vi "layout.vi"(0 "reference":refnum<class "ImplicitParameterNode.lvclass">, 1 "graph":refnum<class "Graph.lvclass">, 2 "graphics":refnum<class "Graphics.lvclass">, 3 "grid":refnum<class "Grid.lvclass">, 5 "error in (no error)":errorcluster) -> (14 "reference out":refnum<class "ImplicitParameterNode.lvclass">, 19 "error out":errorcluster)   [LabVIEW 2014, in "ImplicitParameterNode.lvclass"]
doc: "public void layout(Graph g, Graphics2D g2, Grid grid)"
uses:
  <resource>/Framework/Providers/Open_GDS/UML/ImplicitParameterNode_class/ImplicitParameterNode.lvclass
  <resource>/Framework/Providers/Open_GDS/UML/Graph_class/Graph.lvclass
  <resource>/Framework/Providers/Open_GDS/UML/Graphics_class/Graphics.lvclass
  <resource>/Framework/Providers/Open_GDS/UML/Grid_class/Grid.lvclass
  <resource>/Framework/Providers/Open_GDS/UML/General/Rectangle/Rectangle Rectangle2D.ctl
  <resource>/Framework/Providers/Open_GDS/UML/MultiLineString_class/MultiLineString.lvclass
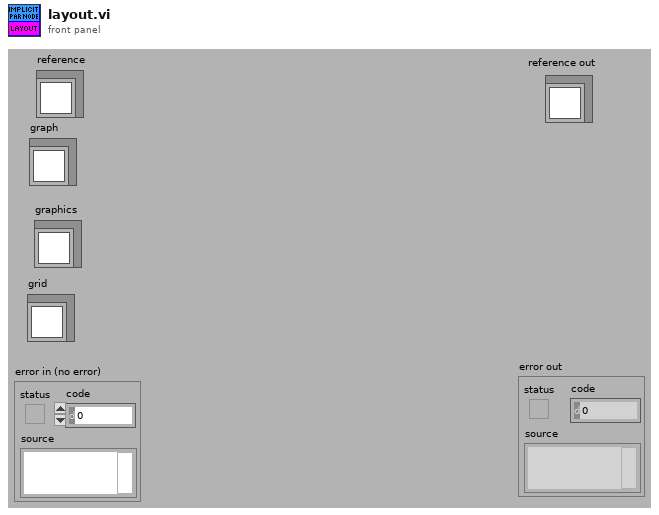
[diagram p1: front panel]
types:
  T1 = typedef "Rectangle Rectangle2D.ctl" = cluster{"x":dbl, "y":dbl, "width":dbl, "height":dbl}
  T2 = typedef "ImplicitParameterNode.lvclass/ObjectAttributes.ctl" = cluster{"Base class":T3, "topHeight":dbl, "name":refnum<class "MultiLineString.lvclass">, "DEFAULT_TOP_HEIGHT":i32, "DEFAULT_WIDTH":i32, "DEFAULT_HEIGHT":i32}
  T3 = typedef "RectangularNode.lvclass/ObjectAttributes.ctl" = cluster{"Base class":T4, "bounds":T1}
  T4 = typedef "AbstractNode.lvclass/ObjectAttributes.ctl" = cluster{"parent":refnum<class "AbstractNode.lvclass">, "children":refnum<class "AbstractNode.lvclass">[], "Hidden":bool}
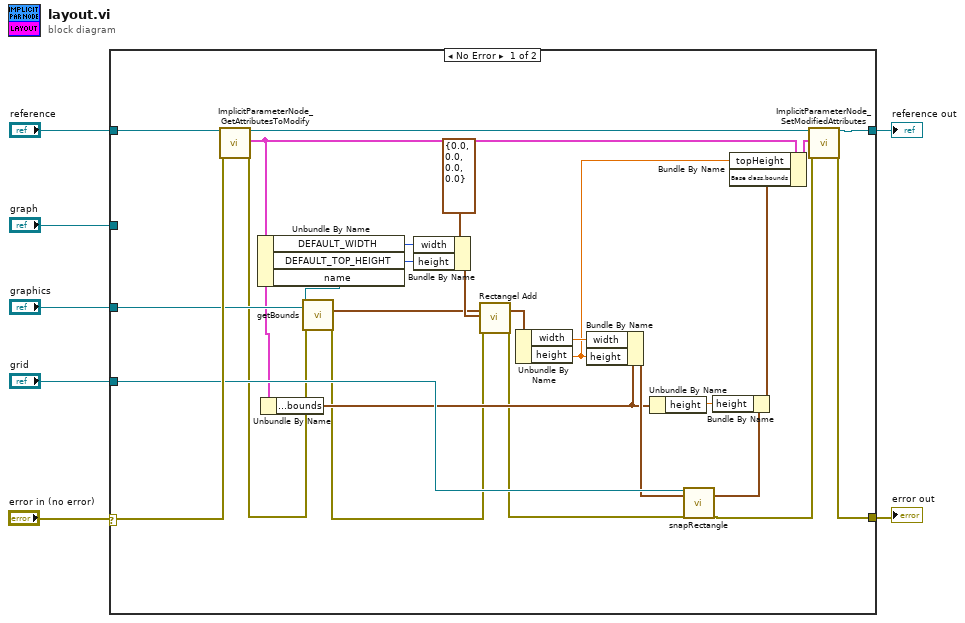
[diagram p0: block diagram]
diagram:
  n1 = case shown="No Error" "error in (no error)" {
    selector: "error in (no error)" -> [w31 w35]
    tunnel: "reference" -> [w34 w36]
    tunnel: [w33 w35] -> w6
    tunnel: [w32 w36] -> w5
    tunnel: "graphics" -> [w30 _]
    tunnel: "grid" -> [w29 _]
    tunnel: "graph" -> [_ _]
    frame No Error {
      n2 = call <resource>:"ImplicitParameterNode_GetAttributesToModify.vi"("reference in"=w34, "error in (no error)"=w31) -> ("reference out"=w28:refnum<class "ImplicitParameterNode.lvclass">, "Attributes"=w15:T2, "error out"=w9:errorcluster)  [unwired: 1 in, 14 out]
      n3 = Unbundle By Name(w15) -> ("DEFAULT_WIDTH"=w25:i32, "DEFAULT_TOP_HEIGHT"=w24:i32, "name"=w26:refnum<class "MultiLineString.lvclass">)
      n4 = Unbundle By Name(w15) -> ("Base class.bounds"=w17:T1)
      n5 = call-dynamic "getBounds.vi"("reference"=w26, "graphics"=w30, "error in (no error)"=w9) -> ("bounds"=w20:T1, "error out"=w10:errorcluster)  [unwired: 15 out]
      n6 = Bundle By Name(cluster=T1 {"x"=0.0, "y"=0.0, "width"=0.0, "height"=0.0} ("bounds"), "width"=w25, "height"=w24) -> (w23:T1)
      n7 = call <resource>:"Rectangel Add.vi"("bounds1"=w20, "bounds2"=w23, "error in (no error)"=w10) -> ("boundsAdded"=w19:T1, "error out"=w11:errorcluster)  [unwired: 2 in, 13 out]
      n8 = Unbundle By Name(w19) -> ("width"=w22:dbl, "height"=w8:dbl)
      n9 = Bundle By Name(cluster=w17, "width"=w22, "height"=w8) -> (w21:T1)
      n10 = Unbundle By Name(w17) -> ("height"=w16:dbl)
      n11 = call <resource>:"snapRectangle.vi"("reference"=w29, "bounds"=w21, "error in (no error)"=w11) -> ("boundsOut"=w18:T1, "error out"=w12:errorcluster)  [unwired: 15 out]
      n12 = Bundle By Name(cluster=w18, "height"=w16) -> (w13:T1)
      n13 = Bundle By Name(cluster=w15, "topHeight"=w8, "Base class.bounds"=w13) -> (w14:T2)
      n14 = call <resource>:"ImplicitParameterNode_SetModifiedAttributes.vi"("reference in"=w28, "Attributes"=w14, "error in (no error)"=w12) -> ("reference out"=w32:refnum<class "ImplicitParameterNode.lvclass">, "error out"=w33:errorcluster)  [unwired: 3 in, 12 out]
    }
    frame Error {
    }
  }
  "reference out" <- w5
  "error out" <- w6
